vi "Contingency Table.vi"(0 "Table":i32[][](array[numeric]) format="%0.0f") -> (1 "x":dbl format="%0.2f", 2 "probability":dbl format="%0.6f", 3 "error":i32)   [LabVIEW 2010, in "NI_AALPro.lvlib"]
doc: "Classifies and tallies objects of experimentation according to two schemes of categorization."
uses:
  NI_AALPro.lvlib
  lvanlys.dll
panel:
  # "Contingency Table"
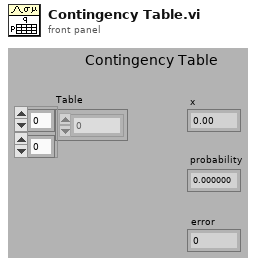
[diagram p1: front panel]
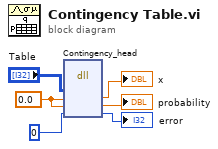
[diagram p0: block diagram]
diagram:
  w4 = 0.0
  n1 = dll-call lib="C:/Program Files/National Instruments/LabVIEW 2010/resource/lvanlys.*" fn="Contingency_head"("Table"="Table", w4, w4, 0) -> (→"x":dbl, →"probability":dbl, →"error":i32)  [unwired: 5 in, 2 out]
